vi "Shapelets Search (GA).vi"() -> ()   [LabVIEW 2016]
uses:
  _vlib/SHAPE_SearchTypes.ctl
  5. Features Optimization/_Optimal Frequency Bands Search/GA_core/GA_tParameters.ctl
  _vlib/SHAPE_AppStates.ctl
  _vlib/Shapelets Search GA.lvclass
  5. Features Optimization/_Optimal Frequency Bands Search/GA_core/GA_tPopulation.ctl
  5. Features Optimization/_Optimal Frequency Bands Search/GA_core/GA_tSolution progress.ctl
  5. Features Optimization/_Optimal Frequency Bands Search/GA_core/GA_tFitness Function.ctl
  Shapelets Search (GA).lvlib
  5. Features Optimization/_Optimal Frequency Bands Search/GA_core/GeneticAlgorithm.lvlib
panel:
  in  "DistanceTable":dbl[][](array[numeric])
  in  "Stop":bool
  out "Application State":string caption="Текущее состояние"
  in  "Tab Control":enum32{"Запуск", "Настройка ГА", "Работа ГА"}(tab)
  in  "Number of Channels":i32=20 caption="Число каналов в записи"
  in  "Next":bool
  in  "Training Data":path caption="Путь к XML-файлу с исходными данными"
  out "Number of Training Trials":i32 caption="Число записей в файле"
  out "Progress":i32(slide) caption="Процесс чтения данных" min=0 max=320 scale=0.0..222.0
  out "TimeSeriesLength":i32 caption="Длина временного ряда"
  in  "ShapeletsNum":i32 caption="Число шейплетов в наборе"
  in  "Parameters":T1={"Population size"=1000, "Generations no."=10, "Significant digits"=4, "Crossover probabality"=0.85, "Mutation mode"=enum."one-point, fixed rate", "Use Gray code?"=TRUE, "Mutation rate"=0.05, "Min mutation rate"=0.0005, "Max mutation rate"=0.25, "Reproduction plan"=enum."Full generational replacement", "Elitism"=TRUE, "Fmax"=1} caption="Параметры генетического алгоритма" {"Max mutation rate" min=0.0 max=1.0; "Min mutation rate" min=0.0 max=1.0; "Mutation rate" min=0.0 max=1.0; "Crossover probabality" min=0.0 max=1.0; "Significant digits" min=1; "Generations no." min=1; "Population size" min=1}
  in  "Start":bool
  in  "Search Type":T2 caption="Тип поиска"
  out "Shapelet Class":string caption="Метка класса"
  out "Shapelet Graph":cluster{i32[], dbl[]}[](graph) caption="Текущий лучший шейплет"
  in  "Set of Shapelets":i32[][](array[numeric]) caption="Итоговый набор шейплетов"
  in  "Solution":i32[][](array[numeric]) caption="Текущее решение на итерациях ГА"
  out "Accuracy Chart":cluster{i32[], dbl[]}[](graph) caption="График функции приспособленности"
  out "Accuracy":dbl caption="Приспособленность"
  out "Generation":i32 caption="Поколение"
  # "This VI is a part of BCI Design library, http://www.ru-bci.org \nCopyright © 2020, Sotnikov Peter, All rights reserved. License: GNU GPLv3"
  # "Входные данные"
  # "Результаты чтения данных"
  # "Размер популяции"
  # "Число поколений"
  # "Вероятность скрещивания (кроссовера)"
  # "Тип мутации"
  # "Вероятность мутации"
  # "Минимальная вероятность мутации"
  # "Максимальная вероятность мутации"
  # "Способ включения потомков в популяцию"
  # "Использовать элитизм?"
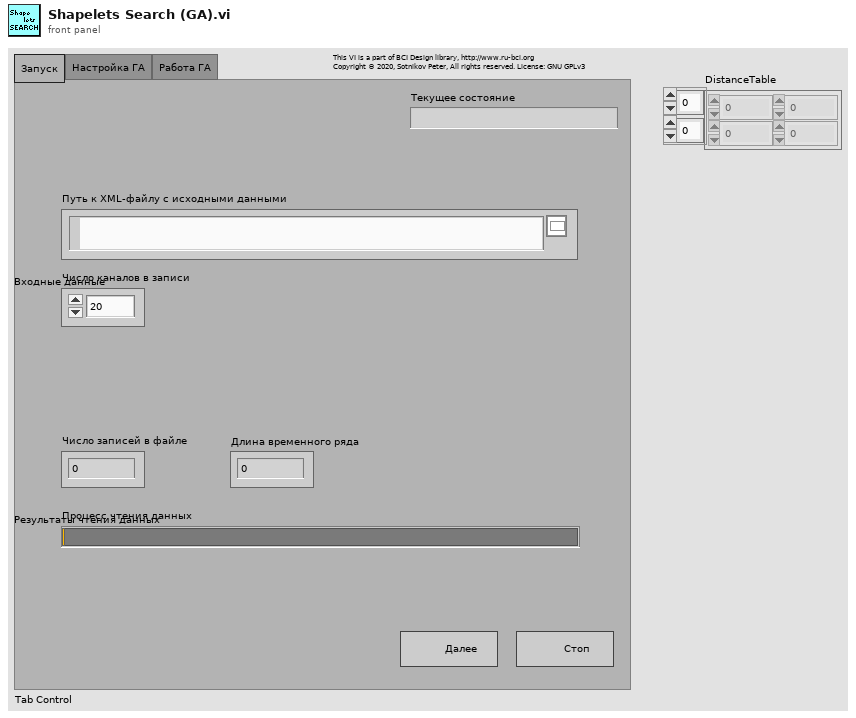
[diagram p1: front panel]
types:
  T1 = typedef "Optimal Frequency Bands Search.lvlib/GeneticAlgorithm.lvlib/GA_tParameters.ctl" = cluster{"Population size":i32, "Generations no.":i32, "Significant digits":i32, "Crossover probabality":dbl, "Mutation mode":enum16{"one-point, fixed rate", "one-point, fitness-adjustable rate", "one-point, distance-adjustable rate"}, "Use Gray code?":bool, "Mutation rate":dbl, "Min mutation rate":dbl, "Max mutation rate":dbl, "Reproduction plan":enum16{"Full generational replacement", "Steady-state-replace-random", "Steady-state-replace-worst"}, "Elitism":bool, "Fmax":i32}
  T2 = typedef "Shapelets Search (GA).lvlib/SHAPE_SearchTypes.ctl" = enum16{"Лучший шейплет", "Набор шейплетов"}
  T3 = typedef "Optimal Frequency Bands Search.lvlib/GeneticAlgorithm.lvlib/GA_tSolution progress.ctl" = cluster{"Solution":i32[], "Fitness":dbl, "Mutation rate":dbl, "Generation":i32}
  T4 = typedef "Optimal Frequency Bands Search.lvlib/GeneticAlgorithm.lvlib/GA_tPopulation.ctl" = cluster{"Population":i32[][], "Fitnesses":dbl[], "Sorted indices":i32[], "Ranks":i32[]}
  T5 = typedef "Shapelets Search (GA).lvlib/SHAPE_AppStates.ctl" = enum16{"Initialize", "ReadTrainData", "ReadTestData", "StartOptimization", "OptimizationProgress", "Stop", "ReInit Optimization"}
  T6 = typedef "Optimal Frequency Bands Search.lvlib/GeneticAlgorithm.lvlib/GA_tFitness Function.ctl" = refnum<vi>
  T7 = cluster{"Number of Training Trials":refnum<vi>, "Progress":refnum<vi>}
  T8 = cluster{"Shapelet":refnum<vi>, "Accuracy":refnum<vi>, "Generation":refnum<vi>, "Solution":refnum<vi>, "Accuracy Chart":refnum<vi>}
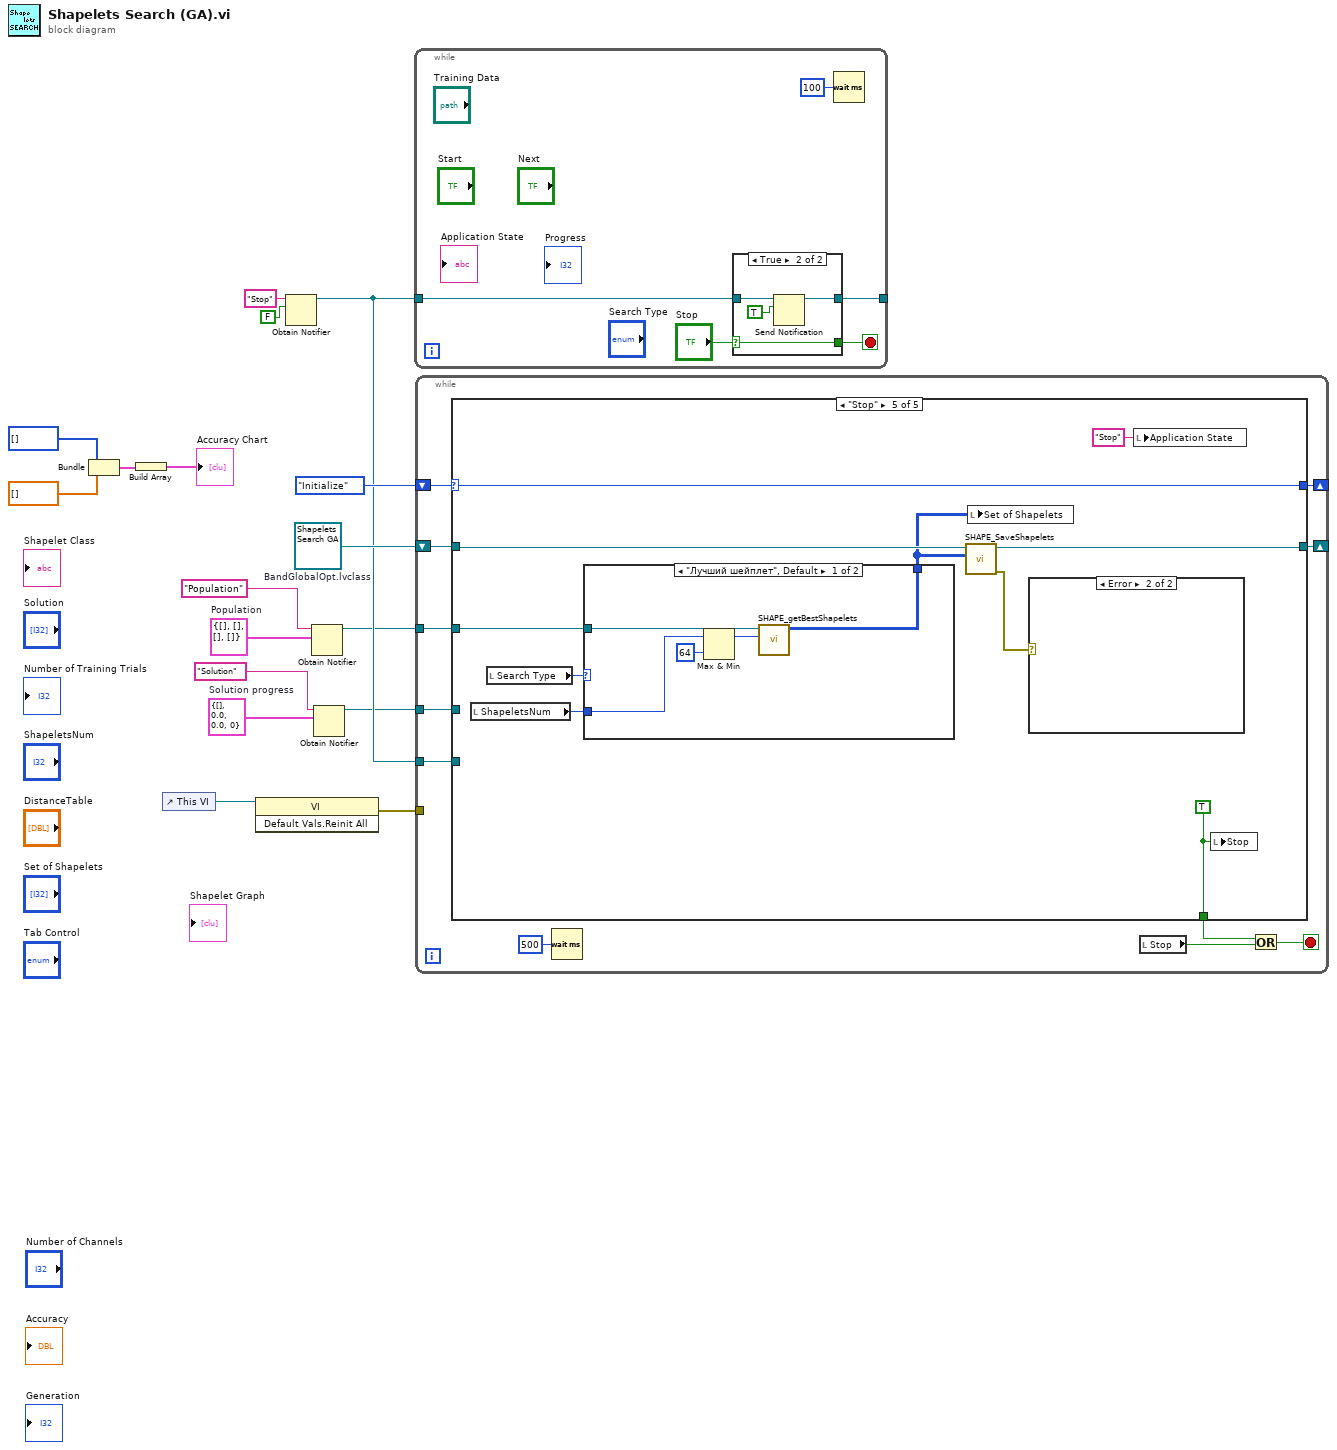
[diagram p0: block diagram]
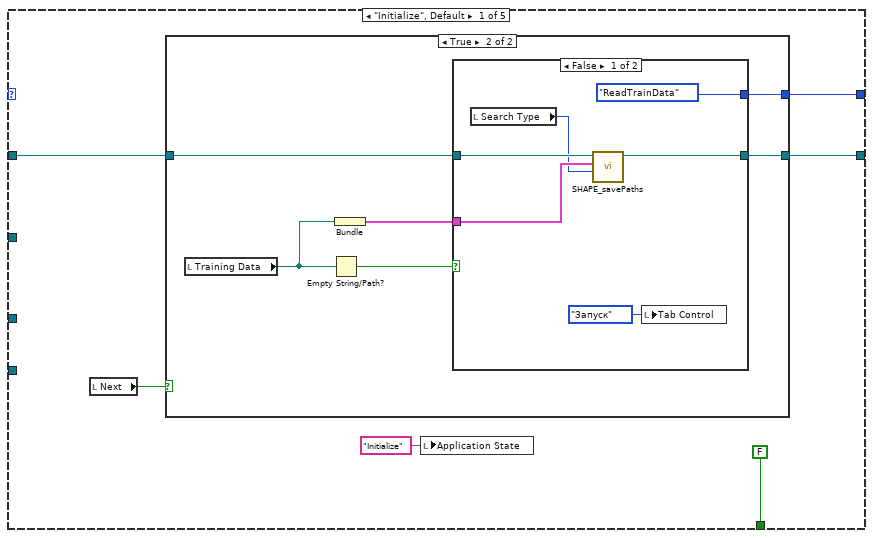
[diagram p3: hidden frame]
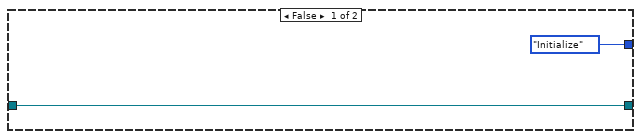
[diagram p4: hidden frame]
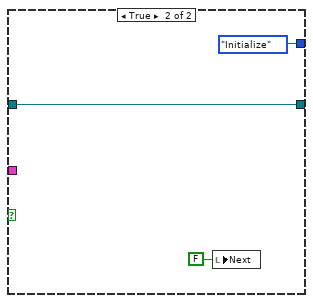
[diagram p5: hidden frame]
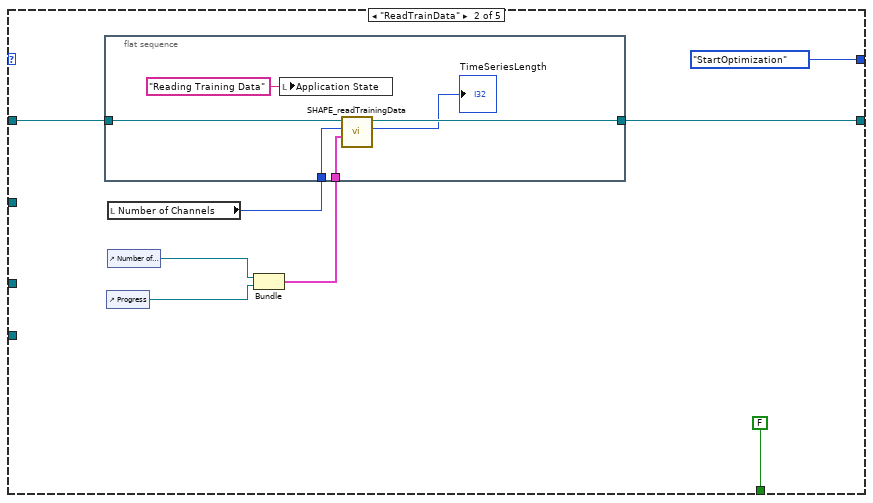
[diagram p6: hidden frame]
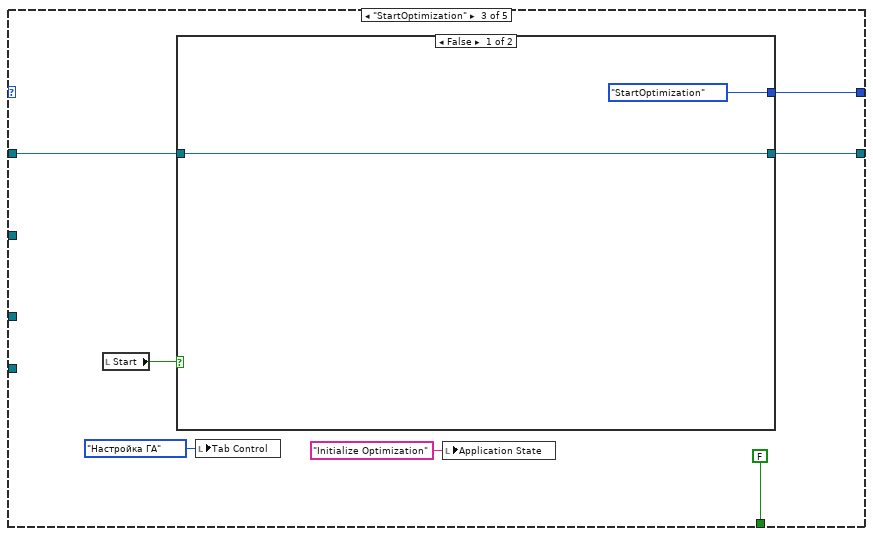
[diagram p7: hidden frame]
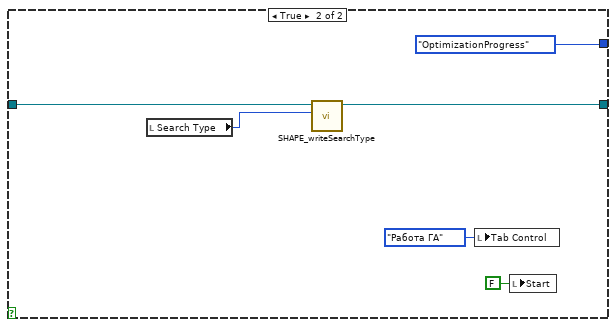
[diagram p8: hidden frame]
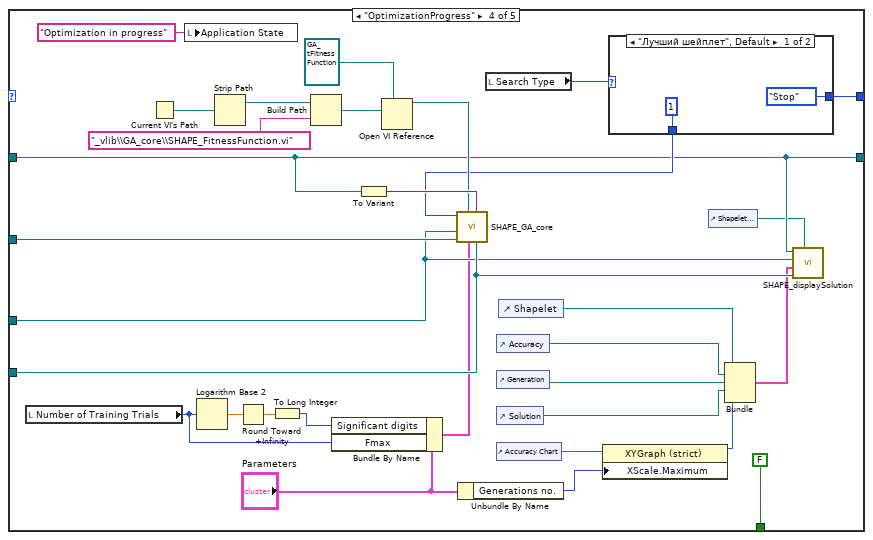
[diagram p9: hidden frame]
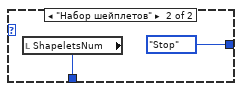
[diagram p10: hidden frame]
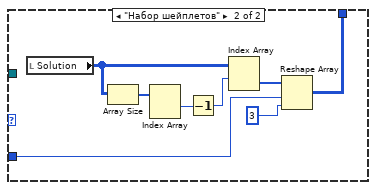
[diagram p11: hidden frame]
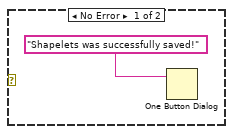
[diagram p12: hidden frame]
diagram:
  w1 = T3 {"Solution"=[], "Fitness"=0.0, "Mutation rate"=0.0, "Generation"=0}  # Solution progress
  w2 = T4 {"Population"=[], "Fitnesses"=[], "Sorted indices"=[], "Ranks"=[]}  # Population
  w16 = refnum<class "Shapelets Search GA.lvclass"> refnum  # BandGlobalOpt.lvclass
  n1 = Bundle(i32[] [], dbl[] []) -> (w8:cluster{i32[], dbl[]})  [unwired: 1 in]
  n2 = Build Array(w8) -> (→"Accuracy Chart":cluster{i32[], dbl[]}[])
  n3 = control-ref of="This VI"() -> (w15:refnum<vi>)
  n4 = invoke class="VI" method="Default Vals.Reinit All"(reference=w15) -> (error out=w14:errorcluster)  [unwired: 2 in, 2 out]
  n5 = Obtain Notifier(name (unnamed)="Stop", notification data type=FALSE) -> (notifier out=w9:refnum<notifier>)  [unwired: 2 in, 2 out]
  n6 = Obtain Notifier(name (unnamed)="Population", notification data type=w2) -> (notifier out=w4:refnum<notifier>)  [unwired: 2 in, 2 out]
  n7 = Obtain Notifier(name (unnamed)="Solution", notification data type=w1) -> (notifier out=w3:refnum<notifier>)  [unwired: 2 in, 2 out]
  n8 = while {
    tunnel: w9 -> [w20]
    tunnel: [w18] -> _
    stop <- w19 stop-if-true
    n9 = case shown="True" "Stop" {
      selector: "Stop" -> [w24 w26]
      tunnel: w20 -> [w23 w28]
      tunnel: [w24 w26] -> w19
      tunnel: [w23 w25] -> w18
      frame False {
      }
      frame True {
        n10 = Send Notification(notification=TRUE, notifier=w28) -> (notifier out=w25:refnum<notifier>)  [unwired: 1 in, 1 out]
      }
    }
    n11 = Wait (ms)(milliseconds to wait=u32 100) -> ()  [unwired: 1 out]
  }
  n12 = while {
    shift-right: [w34] -> _
    shift-left: SHAPE_AppStates."Initialize" ("BGO_AppStates") -> [w39]
    shift-right: [w32] -> _
    shift-left: w16 -> [w33]
    tunnel: w14 -> [_]
    tunnel: w9 -> [w31]
    tunnel: w4 -> [w30]
    tunnel: w3 -> [w29]
    stop <- w38 stop-if-true
    n13 = case shown="\"Stop\"" w39 {
      selector: w39 -> [_ _ _ _ w136]
      tunnel: [FALSE FALSE FALSE FALSE w134] -> w36
      tunnel: [w43 SHAPE_AppStates."StartOptimization" ("BGO_AppStates") w82 w105 w136] -> w34
      tunnel: w33 -> [w42 w66 w80 w94 w130]
      tunnel: [w41 w63 w79 w94 w133] -> w32
      tunnel: w31 -> [_ _ _ w113 _]
      tunnel: w30 -> [_ _ _ w103 w129]
      tunnel: w29 -> [_ _ _ w102 _]
      frame "Initialize", Default {
        n14 = local read "Next"() -> (w45:bool)
        n15 = case shown="True" w45 {
          tunnel: [SHAPE_AppStates."Initialize" ("BGO_AppStates") w53] -> w43
          tunnel: w42 -> [w46 w51]
          tunnel: [w46 w50] -> w41
          frame False {
          }
          frame True {
            n16 = local read "Training Data"() -> (w52:path)
            n17 = Empty String/Path?(string/path=w52) -> (empty?=w48:bool)
            n18 = Bundle("Training Data"=w52) -> (w49:cluster{"Training Data":path})  [unwired: 1 in]
            n19 = case shown="False" w48 {
              tunnel: [SHAPE_AppStates."ReadTrainData" ("BGO_AppStates") SHAPE_AppStates."Initialize" ("BGO_AppStates")] -> w53
              tunnel: w51 -> [w58 w60]
              tunnel: [w57 w60] -> w50
              tunnel: w49 -> [w56 _]
              frame False {
                n20 = local read "Search Type"() -> (w55:T2)
                n21 = call "SHAPE_savePaths.vi"("SearchType"=w55, "Paths"=w56, "BandGlobalOpt in"=w58) -> ("BandGlobalOpt out"=w57:refnum<class "Shapelets Search GA.lvclass">)  [unwired: 7 in, 1 out]
                n22 = local write "Tab Control"(enum32{"Запуск", "Настройка ГА", "Работа ГА"}."Запуск" ("Tab Control")) -> ()
              }
              frame True {
                n23 = local write "Next"(FALSE ("Next")) -> ()
              }
            }
          }
        }
        n24 = local write "Application State"("Initialize" ("Application State")) -> ()
      }
      frame "ReadTrainData" {
        n25 = flat-sequence {
          tunnel: w66 -> [w75]
          tunnel: [w74] -> w63
          tunnel: w65 -> [w73]
          tunnel: w64 -> [w72]
          frame #0 {
            n26 = local write "Application State"("Reading Training Data" ("Application State")) -> ()
            n27 = call "SHAPE_readTrainingData.vi"("ControlRefs"=w73, "NumberOfChannels"=w72, "BandGlobalOpt in"=w75) -> ("TimeSeriesLength"=→"TimeSeriesLength":i32, "BandGlobalOpt out"=w74:refnum<class "Shapelets Search GA.lvclass">)  [unwired: 6 in, 1 out]
          }
        }
        n28 = control-ref of="Progress"() -> (w70:refnum<vi>)
        n29 = local read "Number of Channels"() -> (w64:i32)
        n30 = control-ref of="Number of Training Trials"() -> (w69:refnum<vi>)
        n31 = Bundle("Number of Training Trials"=w69, "Progress"=w70) -> (w65:T7)  [unwired: 1 in]
      }
      frame "StartOptimization" {
        n32 = local read "Start"() -> (w81:bool)
        n33 = case shown="False" w81 {
          tunnel: [SHAPE_AppStates."StartOptimization" ("BGO_AppStates") SHAPE_AppStates."OptimizationProgress" ("BGO_AppStates")] -> w82
          tunnel: w80 -> [w84 w88]
          tunnel: [w84 w87] -> w79
          frame False {
          }
          frame True {
            n34 = local read "Search Type"() -> (w86:T2)
            n35 = call-dynamic "SHAPE_writeSearchType.vi"("Search Type"=w86, "BandGlobalOpt in"=w88) -> ("BandGlobalOpt out"=w87:refnum<class "Shapelets Search GA.lvclass">)  [unwired: 8 in, 1 out]
            n36 = local write "Tab Control"(enum32{"Запуск", "Настройка ГА", "Работа ГА"}."Работа ГА" ("Tab Control")) -> ()
            n37 = local write "Start"(FALSE ("Start")) -> ()
          }
        }
        n38 = local write "Tab Control"(enum32{"Запуск", "Настройка ГА", "Работа ГА"}."Настройка ГА" ("Tab Control")) -> ()
        n39 = local write "Application State"("Initialize Optimization" ("Application State")) -> ()
      }
      frame "OptimizationProgress" {
        n40 = local read "Number of Training Trials"() -> (w93:i32)
        n41 = Current VI's Path() -> (path=w119:path)
        n42 = local write "Application State"("Optimization in progress" ("Application State")) -> ()
        n43 = Logarithm Base 2(1:w93) -> (0:w101:dbl)
        n44 = Strip Path(path=w119) -> (stripped path=w118:path)  [unwired: 1 out]
        n45 = Round Toward +Infinity(x=w101) -> (ceil(x): smallest int >= x=w100:dbl)
        n46 = To Long Integer(number=w100) -> (32bit integer=w99:i32)
        n47 = Build Path(base path=w118, name or relative path="_vlib\\GA_core\\SHAPE_FitnessFunction.vi") -> (appended path=w116:path)
        n48 = Bundle By Name(cluster="Parameters", "Significant digits"=w99, "Fmax"=w93) -> (w98:T1)
        n49 = To Variant(anything=w94) -> (Variant=w120:variant)
        n50 = Open VI Reference(type specifier VI Refnum (for type only)=T6 refnum ("Fitness Function"), vi path=w116) -> (vi reference=w114:T6)  [unwired: 4 in, 1 out]
        n51 = Unbundle By Name("Parameters") -> ("Generations no."=w96:i32)
        n52 = local read "Search Type"() -> (w106:T2)
        n53 = control-ref of="Accuracy"() -> (w112:refnum<vi>)
        n54 = control-ref of="Generation"() -> (w111:refnum<vi>)
        n55 = control-ref of="Solution"() -> (w110:refnum<vi>)
        n56 = control-ref of="Accuracy Chart"() -> (w109:refnum<vi>)
        n57 = control-ref of="Shapelet"() -> (w95:refnum<vi>)
        n58 = property class="XYGraph (strict)"(reference=w109, "XScale.Maximum"=w96) -> (reference out=w108:refnum<vi>)  [unwired: 1 in, 1 out]
        n59 = case shown="\"Лучший шейплет\", Default" w106 {
          tunnel: [SHAPE_AppStates."Stop" ("BGO_AppStates") SHAPE_AppStates."Stop" ("BGO_AppStates")] -> w105
          tunnel: [1 ("Phenotype size") w125] -> w104
          frame "Лучший шейплет", Default {
          }
          frame "Набор шейплетов" {
            n60 = local read "ShapeletsNum"() -> (w125:i32)
          }
        }
        n61 = call "SHAPE_GA_core.vi"("Stop notifier"=w113, "Fitness Function Data"=w120, "Parameters"=w98, "Fitness Function"=w114, "Population notifier"=w103, "Solution Progress notifier"=w102, "Phenotype size"=w104) -> ()  [unwired: 2 in, 3 out]
        n62 = control-ref of="Shapelet Class"() -> (w92:refnum<vi>)
        n63 = Bundle("Shapelet"=w95, "Accuracy"=w112, "Generation"=w111, "Solution"=w110, "Accuracy Chart"=w108) -> (w107:T8)  [unwired: 1 in]
        n64 = call "SHAPE_displaySolution.vi"("Class Label"=w92, "Stop Notifier In"=w113, "Control Refs"=w107, "Solution notifier"=w102, "BandGlobalOpt.lvclass"=w94) -> ()  [unwired: 7 in]
      }
      frame "Stop" {
        w134 = TRUE
        n65 = local read "ShapeletsNum"() -> (w127:i32)
        n66 = local read "Search Type"() -> (w131:T2)
        n67 = case shown="\"Лучший шейплет\", Default" w131 {
          tunnel: [w140 w146] -> w128
          tunnel: w129 -> [w141 _]
          tunnel: w127 -> [w139 w142]
          frame "Лучший шейплет", Default {
            n68 = Max & Min(x=w139, y=64) -> (max(x,y)=w137:i32)  [unwired: 1 out]
            n69 = call "SHAPE_getBestShapelets.vi"("Number of Shapelets"=w137, "Population Notifier"=w141) -> ("Population out"=w140:i32[][])  [unwired: 9 in]
          }
          frame "Набор шейплетов" {
            n70 = local read "Solution"() -> (w145:i32[][])
            n71 = Array Size(array=w145) -> (size(s)=w149:i32[])
            n72 = Index Array(array=w149) -> (element #1=w148:i32)  [unwired: 2 in, 1 out]
            n73 = Decrement(x=w148) -> (x-1=w144:i32)
            n74 = Index Array(array=w145, index (row)=w144) -> (element=w143:i32[])  [unwired: 1 in]
            n75 = Reshape Array(w143, w142, 3 ("dimension size")) -> (w146:i32[][])
          }
        }
        n76 = call "SHAPE_SaveShapelets.vi"("Set of Shapelets"=w128, "BandGlobalOpt in"=w130) -> ("error out"=w132:errorcluster, "BandGlobalOpt out"=w133:refnum<class "Shapelets Search GA.lvclass">)  [unwired: 7 in, 1 out]
        n77 = local write "Set of Shapelets"(w128) -> ()
        n78 = case shown="Error" w132 {
          frame No Error {
            n79 = One Button Dialog(message="Shapelets was successfully saved!") -> ()  [unwired: 1 in, 1 out]
          }
          frame Error {
          }
        }
        n80 = local write "Application State"("Stop" ("Application State")) -> ()
        n81 = local write "Stop"(w134) -> ()
      }
    }
    n82 = Wait (ms)(milliseconds to wait=u32 500) -> ()  [unwired: 1 out]
    n83 = local read "Stop"() -> (w37:bool)
    n84 = Or(x=w36, y=w37) -> (x .or. y?=w38:bool)
  }
